vi "DAQgates.vi"() -> ()   [LabVIEW 2013]
uses:
  <vilib>/DAQmx/read.llb/DAQmx Read (Analog 1D DBL NChan 1Samp).vi
  <vilib>/DAQmx/create/channels.llb/DAQmx Create Channel (AI-Voltage-Basic).vi
  <vilib>/DAQmx/miscellaneous.llb/DAQmx Fill In Error Info.vi
panel:
  in  "Quick Sym val":dbl=5.0 format="%#_13g"
  in  "Both":bool=TRUE
  out "error out 2":errorcluster
  in  "Write 2":bool
  in  "Write 1":bool
  out "AO 1 read":dbl=-0.0007450332912376145
  out "AO 0 read":dbl=-0.0004227007909203878
  in  "Go":bool
  in  "Static Channels 2":cluster{dbl, string, "Output Channels":tag}[](array[cluster])=[{1.0, "", "Output Channels"="Dev3/ao0"}, {1.0, "", "Output Channels"="Dev3/ao1"}, {1.0, "", "Output Channels"="Dev2/ao2"}, {1.0, "", "Output Channels"="Dev2/ao3"}, {0.0, "", "Output Channels"=""}, {1.0, "", "Output Channels"=""}]
  in  "Quick sym -+":bool
  in  "Quick sym +-":bool
  in  "Zero":bool
  in  "AO 1 Write":dbl
  in  "Step Time(s)":dbl=0.05
  in  "Step size(V)":dbl=0.025
  in  "AO 0 Write":dbl
  in  "delay before read (ms)":u32=500
  in  "stop":bool=TRUE
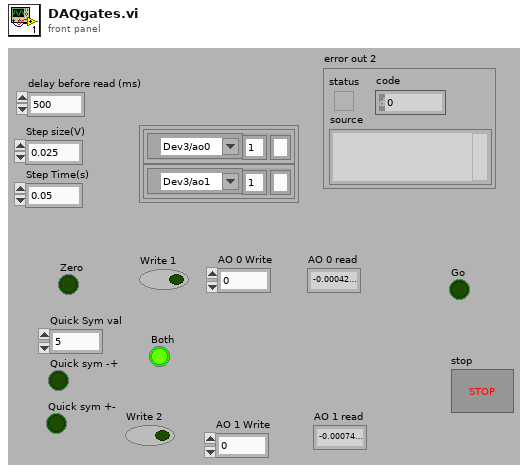
[diagram p1: front panel]
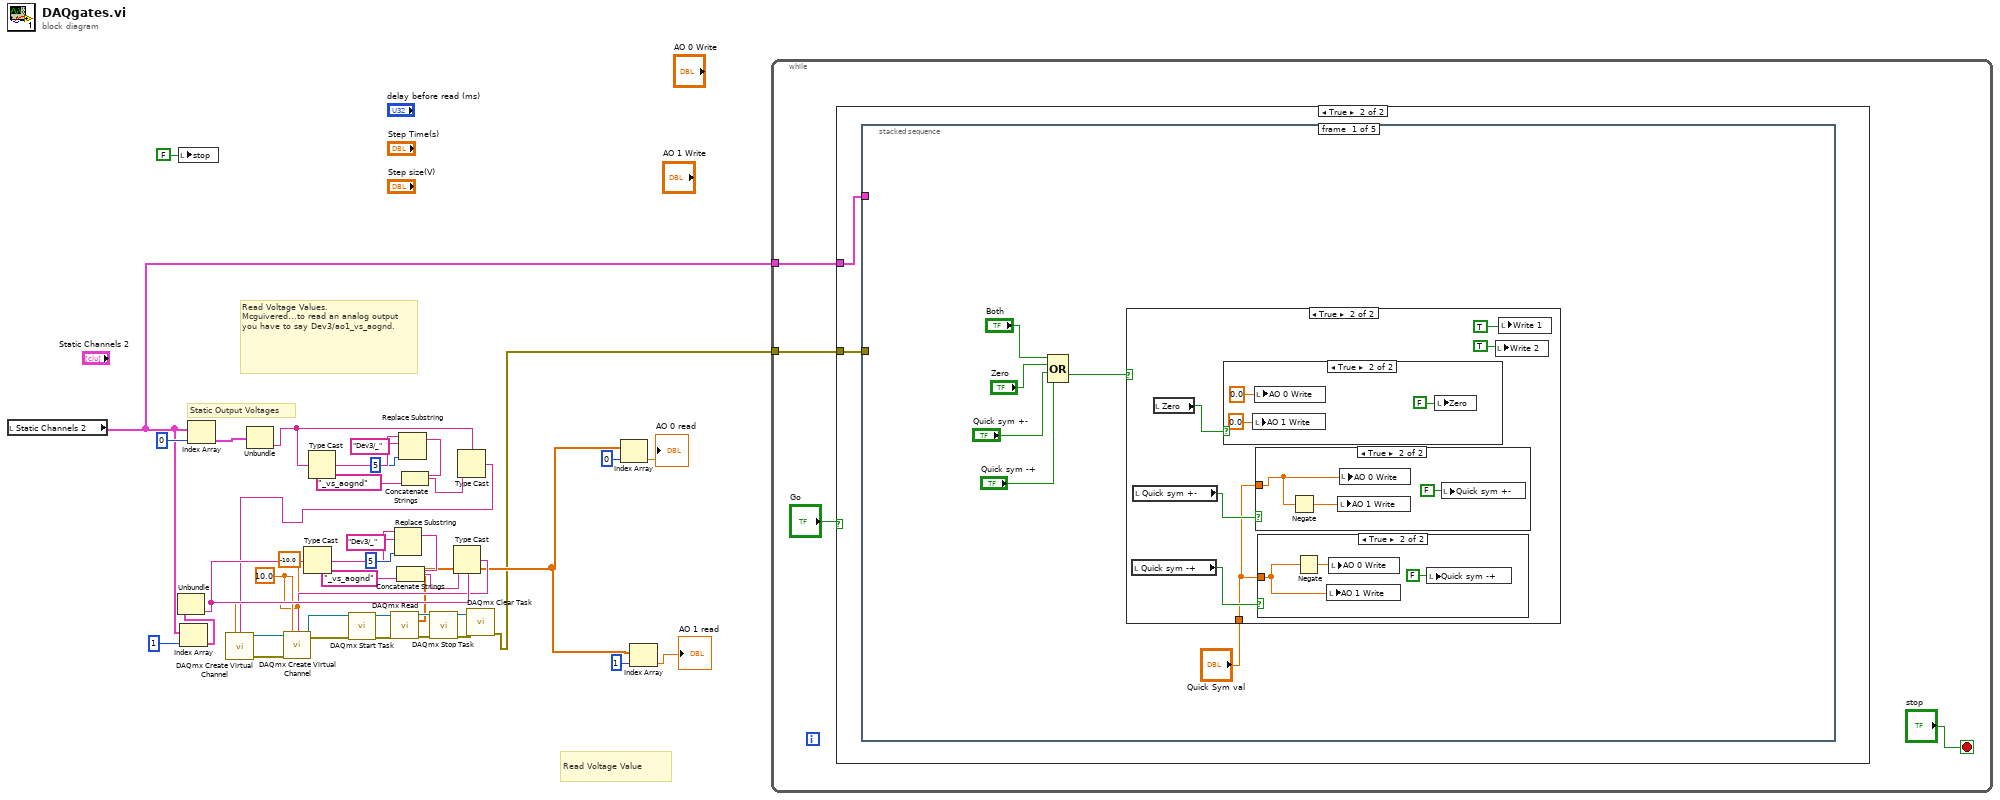
[diagram p0: block diagram]
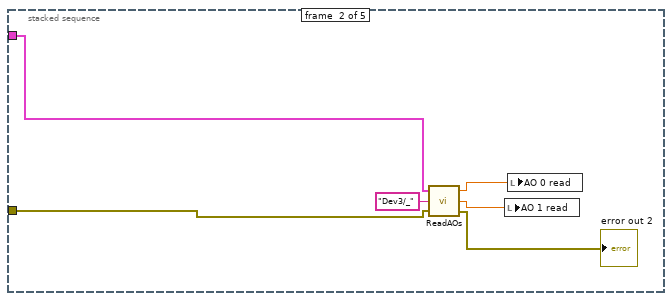
[diagram p7: hidden frame]
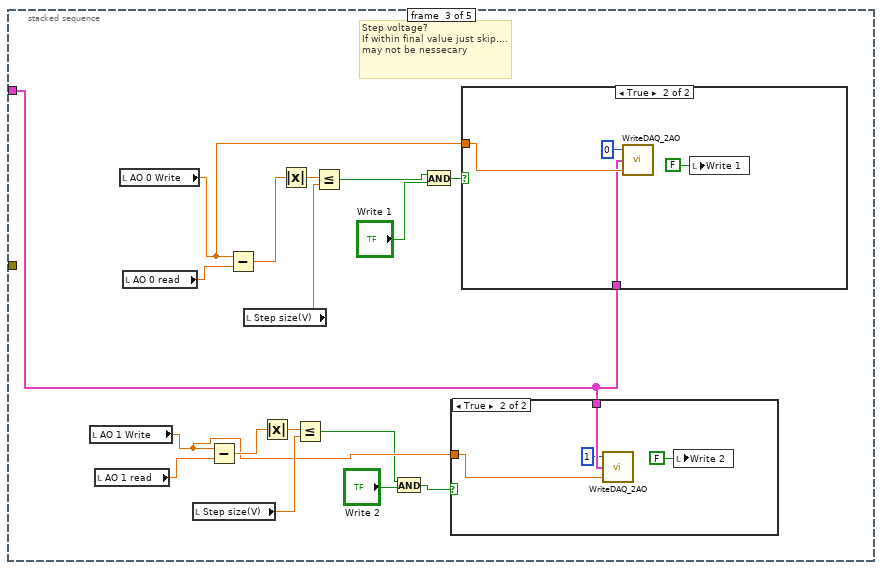
[diagram p8: hidden frame]
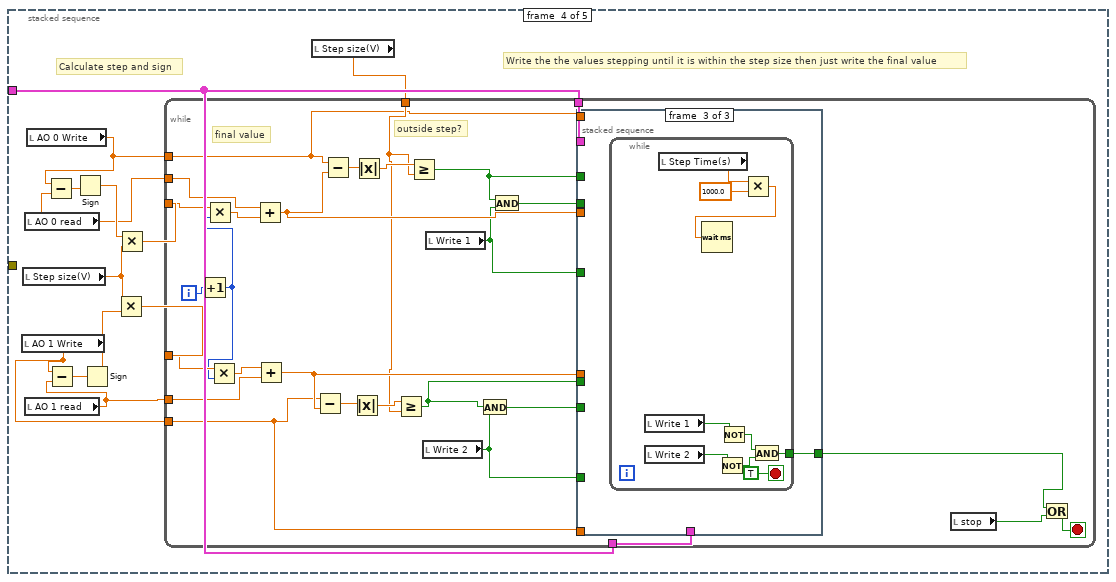
[diagram p11: hidden frame]
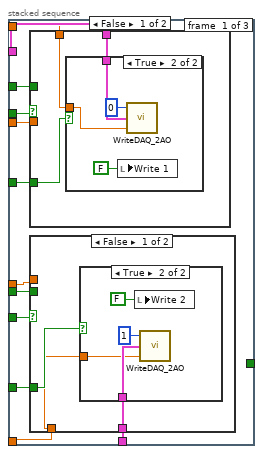
[diagram p12: hidden frame]
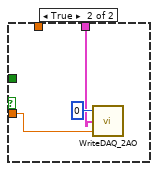
[diagram p14: hidden frame]
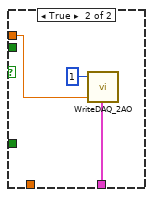
[diagram p16: hidden frame]
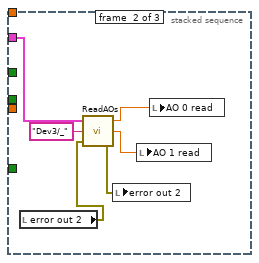
[diagram p17: hidden frame]
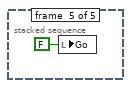
[diagram p18: hidden frame]
diagram:
  w13 = -10.0 ("minimum value")
  w14 = 10.0 ("maximum value")
  # "Static Output Voltages"
  # "Read Voltage Value"
  # "Read Voltage Values. \nMcguivered...to read an analog output you have to say Dev3/ao1_vs_aognd."
  n1 = local read "Static Channels 2"() -> (w5:cluster{dbl, string, "Output Channels":tag}[])
  n2 = local write "stop"(FALSE ("stop")) -> ()
  n3 = Index Array(array=w5, index=1) -> (element=w39:cluster{dbl, string, "Output Channels":tag})
  n4 = Unbundle(w39) -> ("Output Channels"=w28:tag)  [unwired: 2 out]
  n5 = Index Array(array=w5, index=0) -> (element=w40:cluster{dbl, string, "Output Channels":tag})
  n6 = Unbundle(w40) -> ("Output Channels"=w21:tag)  [unwired: 2 out]
  n7 = Type Cast(x=w28) -> (*(type *) &x=w31:string)  [unwired: 1 in]
  n8 = Type Cast(x=w21) -> (*(type *) &x=w27:string)  [unwired: 1 in]
  n9 = Replace Substring(2:5 ("length (len. of substring)"), 4:"Dev3/_" ("substring (\"\")"), 5:w31) -> (1:w34:string)  [unwired: 1 in, 1 out]
  n10 = Concatenate Strings(w34, "_vs_aognd" ("string")) -> (w36:string)
  n11 = Replace Substring(2:5 ("length (len. of substring)"), 4:"Dev3/_" ("substring (\"\")"), 5:w27) -> (1:w24:string)  [unwired: 1 in, 1 out]
  n12 = Concatenate Strings(w24, "_vs_aognd" ("string")) -> (w22:string)
  n13 = Type Cast(type=w28, x=w36) -> (*(type *) &x=w18:tag)
  n14 = Type Cast(type=w21, x=w22) -> (*(type *) &x=w20:tag)
  n15 = call-poly <vilib>:"DAQmx Create Virtual Channel.vi"("maximum value"=w14, "minimum value"=w13, "physical channels"=w20) -> ("task out"=w19:refnum<k21>, "error out"=w15:errorcluster)  [unwired: 11 in]
  n16 = call-poly <vilib>:"DAQmx Create Virtual Channel.vi"("task in"=w19, "maximum value"=w14, "minimum value"=w13, "physical channels"=w18, "error in"=w15) -> ("task out"=w10:refnum<k21>, "error out"=w9:errorcluster)  [unwired: 9 in]
  n17 = call <vilib>:"DAQmx Start Task.vi"("task/channels in"=w10, "error in"=w9) -> ("task out"=w12:refnum<k21>, "error out"=w11:errorcluster)  [unwired: 12 in]
  n18 = call-poly <vilib>:"DAQmx Read.vi"("task/channels in"=w12, "error in"=w11) -> ("task out"=w29:refnum<k21>, "data"=w6:dbl[], "error out"=w16:errorcluster)  [unwired: 11 in]
  n19 = call <vilib>:"DAQmx Stop Task.vi"("task/channels in"=w29, "error in"=w16) -> ("task out"=w30:refnum<k21>, "error out"=w17:errorcluster)  [unwired: 12 in]
  n20 = call <vilib>:"DAQmx Clear Task.vi"("task in"=w30, "error in"=w17) -> ("error out"=w4:errorcluster)  [unwired: 13 in]
  n21 = Index Array(array=w6, index=0) -> (element=→"AO 0 read":dbl)
  n22 = Index Array(array=w6, index=1) -> (element=→"AO 1 read":dbl)
  n23 = while {
    tunnel: w5 -> [w42]
    tunnel: w4 -> [w41]
    stop <- "stop" stop-if-true
    n24 = case shown="True" "Go" {
      tunnel: w42 -> [_ w46]
      tunnel: w41 -> [_ w45]
      frame False {
      }
      frame True {
        n25 = stacked-sequence {
          tunnel: w46 -> [_ w70 w80 w111 _]
          tunnel: w45 -> [_ w69 _ _ _]
          frame #0 {
            n26 = Compound Arithmetic op=OR("Both", "Zero", "Quick sym +-", "Quick sym -+") -> (w49:bool)
            n27 = case shown="True" w49 {
              tunnel: "Quick Sym val" -> [_ w53]
              frame False {
              }
              frame True {
                n28 = local read "Quick sym -+"() -> (w56:bool)
                n29 = local read "Quick sym +-"() -> (w57:bool)
                n30 = local read "Zero"() -> (w58:bool)
                n31 = case shown="True" w58 {
                  frame False {
                  }
                  frame True {
                    n32 = local write "AO 1 Write"(0.0 ("Aux 2 Write")) -> ()
                    n33 = local write "AO 0 Write"(0.0 ("Aux 1 Write")) -> ()
                    n34 = local write "Zero"(FALSE ("Zero")) -> ()
                  }
                }
                n35 = case shown="True" w57 {
                  tunnel: w53 -> [_ w62]
                  frame False {
                  }
                  frame True {
                    n36 = Negate(x=w62) -> (-x=w63:dbl)
                    n37 = local write "AO 1 Write"(w63) -> ()
                    n38 = local write "AO 0 Write"(w62) -> ()
                    n39 = local write "Quick sym +-"(FALSE ("1= +10 2=-10")) -> ()
                  }
                }
                n40 = case shown="True" w56 {
                  tunnel: w53 -> [_ w60]
                  frame False {
                  }
                  frame True {
                    n41 = Negate(x=w60) -> (-x=w59:dbl)
                    n42 = local write "AO 1 Write"(w60) -> ()
                    n43 = local write "AO 0 Write"(w59) -> ()
                    n44 = local write "Quick sym -+"(FALSE ("1= -10 2=+10")) -> ()
                  }
                }
                n45 = local write "Write 2"(TRUE ("Write 2")) -> ()
                n46 = local write "Write 1"(TRUE ("Write 1")) -> ()
              }
            }
          }
          frame #1 {
            n47 = call "ReadAOs.vi"("error in"=w69, "substring (\"\")"="Dev3/_" ("substring (\"\")"), "array"=w70) -> ("error out 2"=→"error out 2":errorcluster, "AO1"=w72:dbl, "AO0"=w73:dbl)
            n48 = local write "AO 1 read"(w72) -> ()
            n49 = local write "AO 0 read"(w73) -> ()
          }
          frame #2 {
            # "Step voltage?\nIf within final value just skip....may not be nessecary"
            n50 = local read "AO 1 Write"() -> (w82:dbl)
            n51 = local read "AO 1 read"() -> (w83:dbl)
            n52 = local read "AO 0 Write"() -> (w81:dbl)
            n53 = local read "AO 0 read"() -> (w87:dbl)
            n54 = local read "Step size(V)"() -> (w84:dbl)
            n55 = Subtract(x=w82, y=w83) -> (x-y=w86:dbl)
            n56 = Subtract(x=w81, y=w87) -> (x-y=w89:dbl)
            n57 = local read "Step size(V)"() -> (w88:dbl)
            n58 = Absolute Value(x=w86) -> (abs(x)=w85:dbl)
            n59 = Absolute Value(x=w89) -> (abs(x)=w90:dbl)
            n60 = Less Or Equal?(x=w85, y=w84) -> (x <= y?=w75:bool)
            n61 = Less Or Equal?(x=w90, y=w88) -> (x <= y?=w78:bool)
            n62 = And(x=w75, y="Write 2") -> (x .and. y?=w74:bool)
            n63 = And(x=w78, y="Write 1") -> (x .and. y?=w79:bool)
            n64 = case shown="True" w74 {
              tunnel: w82 -> [_ w94]
              tunnel: w80 -> [_ w93]
              frame False {
              }
              frame True {
                n65 = call "WriteDAQ_2AO.vi"("data"=w94, "array"=w93, "Channel"=1) -> ()
                n66 = local write "Write 2"(FALSE ("Write 1")) -> ()
              }
            }
            n67 = case shown="True" w79 {
              tunnel: w81 -> [_ w98]
              tunnel: w80 -> [_ w96]
              frame False {
              }
              frame True {
                n68 = call "WriteDAQ_2AO.vi"("data"=w98, "array"=w96, "Channel"=0) -> ()
                n69 = local write "Write 1"(FALSE ("Write 1")) -> ()
              }
            }
          }
          frame #3 {
            # "Calculate step and sign"
            # "Write the the values stepping until it is within the step size then just write the final value"
            n70 = local read "AO 1 Write"() -> (w99:dbl)
            n71 = local read "Step size(V)"() -> (w107:dbl)
            n72 = local read "AO 0 read"() -> (w103:dbl)
            n73 = local read "AO 1 read"() -> (w102:dbl)
            n74 = local read "AO 0 Write"() -> (w101:dbl)
            n75 = Subtract(x=w101, y=w103) -> (x-y=w109:dbl)
            n76 = Subtract(x=w99, y=w102) -> (x-y=w110:dbl)
            n77 = Sign(1:w109) -> (0:w108:dbl)
            n78 = Sign(1:w110) -> (0:w106:dbl)
            n79 = Multiply(x=w107, y=w106) -> (x*y=w104:dbl)
            n80 = Multiply(x=w108, y=w107) -> (x*y=w105:dbl)
            n81 = local read "Step size(V)"() -> (w100:dbl)
            n82 = while {
              tunnel: w111 -> [w125]
              tunnel: w111 -> [w124]
              tunnel: w105 -> [w120]
              tunnel: w104 -> [w123]
              tunnel: w103 -> [w119]
              tunnel: w102 -> [w117]
              tunnel: w101 -> [w114]
              tunnel: w100 -> [w115]
              tunnel: w99 -> [w113]
              i -> [w122]
              stop <- w129 stop-if-true
              # "outside step?"
              # "final value"
              n83 = Increment(x=w122) -> (x+1=w121:i32)
              n84 = Multiply(x=w120, y=w121) -> (x*y=w118:dbl)
              n85 = Multiply(x=w123, y=w121) -> (x*y=w116:dbl)
              n86 = Add(x=w119, y=w118) -> (x+y=w132:dbl)
              n87 = Add(x=w116, y=w117) -> (x+y=w137:dbl)
              n88 = Subtract(x=w113, y=w137) -> (x-y=w138:dbl)
              n89 = Subtract(x=w114, y=w132) -> (x-y=w131:dbl)
              n90 = Absolute Value(x=w138) -> (abs(x)=w139:dbl)
              n91 = Absolute Value(x=w131) -> (abs(x)=w130:dbl)
              n92 = Greater Or Equal?(x=w139, y=w115) -> (x >= y?=w135:bool)
              n93 = Greater Or Equal?(x=w130, y=w115) -> (x >= y?=w134:bool)
              n94 = local read "Write 2"() -> (w126:bool)
              n95 = local read "Write 1"() -> (w127:bool)
              n96 = And(x=w135, y=w126) -> (x .and. y?=w136:bool)
              n97 = And(x=w134, y=w127) -> (x .and. y?=w133:bool)
              n98 = stacked-sequence {
                tunnel: w137 -> [w151 _ _]
                tunnel: w136 -> [w150 _ _]
                tunnel: w135 -> [w149 _ _]
                tunnel: w134 -> [w148 _ _]
                tunnel: w133 -> [w147 _ _]
                tunnel: w132 -> [w146 _ _]
                tunnel: w127 -> [w145 _ _]
                tunnel: w126 -> [w144 _ _]
                tunnel: w125 -> [w143 w174 _]
                tunnel: w124 -> [w142 _ _]
                tunnel: w114 -> [w141 _ _]
                tunnel: w113 -> [w140 _ _]
                tunnel: [_ _ w178] -> w112
                frame #0 {
                  n99 = case shown="False" w147 {
                    tunnel: w146 -> [_ w160]
                    tunnel: w148 -> [_ _]
                    tunnel: w145 -> [w154 _]
                    tunnel: w141 -> [w153 _]
                    tunnel: w143 -> [w152 w159]
                    frame False {
                      n100 = case shown="True" w154 {
                        tunnel: w153 -> [_ w156]
                        tunnel: w152 -> [_ w158]
                        frame False {
                        }
                        frame True {
                          n101 = local write "Write 1"(FALSE ("Write 1")) -> ()
                          n102 = call "WriteDAQ_2AO.vi"("data"=w156, "array"=w158, "Channel"=0) -> ()
                        }
                      }
                    }
                    frame True {
                      n103 = call "WriteDAQ_2AO.vi"("data"=w160, "array"=w159, "Channel"=0) -> ()
                    }
                  }
                  n104 = case shown="False" w150 {
                    tunnel: w151 -> [_ w169]
                    tunnel: w149 -> [_ _]
                    tunnel: w144 -> [w164 _]
                    tunnel: w140 -> [w163 _]
                    tunnel: w142 -> [w162 w171]
                    frame False {
                      n105 = case shown="True" w164 {
                        tunnel: w163 -> [_ w166]
                        tunnel: w162 -> [_ w168]
                        frame False {
                        }
                        frame True {
                          n106 = local write "Write 2"(FALSE ("Write 2")) -> ()
                          n107 = call "WriteDAQ_2AO.vi"("data"=w166, "array"=w168, "Channel"=1) -> ()
                        }
                      }
                    }
                    frame True {
                      n108 = call "WriteDAQ_2AO.vi"("data"=w169, "array"=w171, "Channel"=1) -> ()
                    }
                  }
                }
                frame #1 {
                  n109 = local read "error out 2"() -> (w172:errorcluster)
                  n110 = call "ReadAOs.vi"("error in"=w172, "substring (\"\")"="Dev3/_" ("substring (\"\")"), "array"=w174) -> ("error out 2"=w175:errorcluster, "AO1"=w176:dbl, "AO0"=w177:dbl)
                  n111 = local write "error out 2"(w175) -> ()
                  n112 = local write "AO 1 read"(w176) -> ()
                  n113 = local write "AO 0 read"(w177) -> ()
                }
                frame #2 {
                  n114 = while {
                    tunnel: [w183] -> w178
                    stop <- TRUE stop-if-true
                    n115 = local read "Write 1"() -> (w187:bool)
                    n116 = local read "Write 2"() -> (w186:bool)
                    n117 = local read "Step Time(s)"() -> (w181:dbl)
                    n118 = Not(x=w186) -> (.not. x?=w184:bool)
                    n119 = Not(x=w187) -> (.not. x?=w185:bool)
                    n120 = Multiply(x=w181, y=1000.0) -> (x*y=w180:dbl)
                    n121 = Wait (ms)(milliseconds to wait=w180) -> ()  [unwired: 1 out]
                    n122 = And(x=w185, y=w184) -> (x .and. y?=w183:bool)
                  }
                }
              }
              n123 = local read "stop"() -> (w128:bool)
              n124 = Or(x=w112, y=w128) -> (x .or. y?=w129:bool)
            }
          }
          frame #4 {
            n125 = local write "Go"(FALSE ("Go")) -> ()
          }
        }
      }
    }
  }
